vi "字符串转数组.vi"(11 "输入字符串":string) -> (1 "解析后布尔数组":bool[](array[boolean]), 2 "解析后数值数组":i32[](array[numeric]), 3 "解析后字符数组":string[](array[string]))   [LabVIEW 2017]
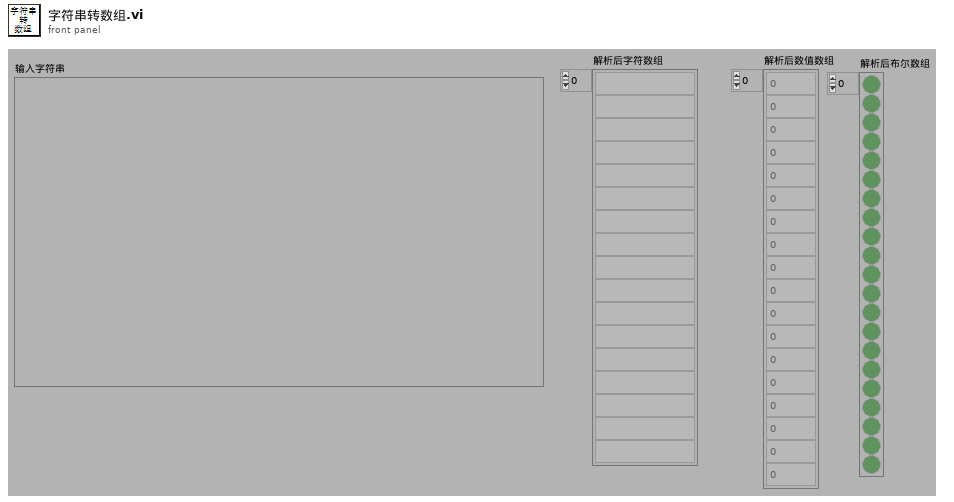
[diagram p1: front panel]
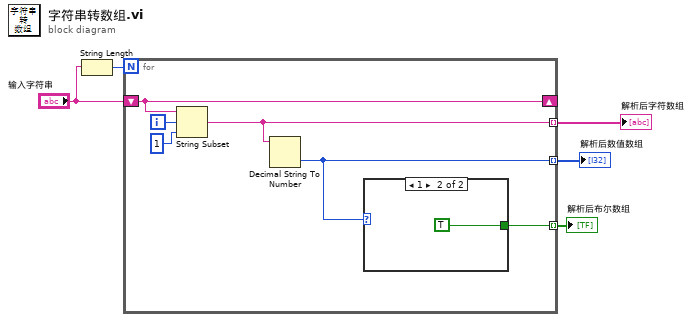
[diagram p0: block diagram]
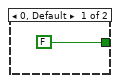
[diagram p2: hidden frame]
diagram:
  n1 = String Length(string="输入字符串") -> (length=w4:i32)
  n2 = for {
    N: w4 -> [_]
    shift-right: [w9] -> _
    shift-left: "输入字符串" -> [w9]
    tunnel: [w8] -> w5 mode=indexing
    tunnel: [w7] -> w2 mode=indexing
    tunnel: [w6] -> w1 mode=indexing
    i -> [w11]
    n3 = String Subset(string=w9, offset (0)=w11, length (rest)=1 ("长度（剩余）")) -> (substring=w8:string)
    n4 = Decimal String To Number(string=w8) -> (number=w7:i32)  [unwired: 2 in, 1 out]
    n5 = case shown="1" w7 {
      tunnel: [FALSE TRUE] -> w6
      frame 0, Default {
      }
      frame 1 {
      }
    }
  }
  "解析后字符数组" <- w5
  "解析后数值数组" <- w2
  "解析后布尔数组" <- w1
